vi "UpdateChannelsList.vi"(8 "error in (no error)":errorcluster, 9 "channels":string[](array[string]), 10 "asset code":string, 11 "ByteQXAPIBase in":refnum<class "ByteQXAPIBase.lvclass">) -> (0 "error out":errorcluster, 3 "ByteQXAPIBase out":refnum<class "ByteQXAPIBase.lvclass">)   [LabVIEW 2019, in "ByteQXWebAPI.lvlib" / "ByteQXAPIBase.lvclass"]
doc: "Sends the asset's available channels list"
uses:
  ByteQXAPIBase.lvclass
  Private/module.ctl
  ChannelsList_ReqData.ctl
  ByteQXAPIBase.lvclass/ByteQXAPIBase.ctl
  <vilib>/Bytelabs/ByteREST/ByteRESTClass/ByteRESTBase/RESTBase.lvclass
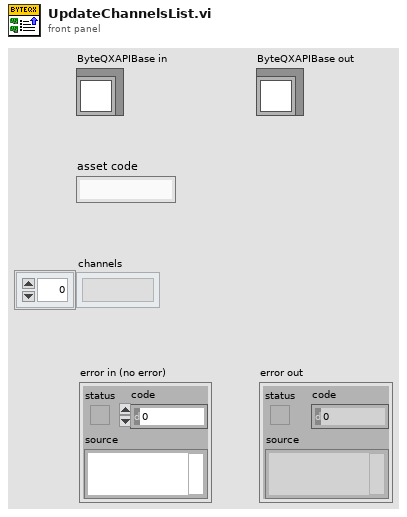
[diagram p1: front panel]
types:
  T1 = typedef "ByteQXWebAPI.lvlib/ByteQXAPIBase.lvclass/ChannelsList_ReqData.ctl" = cluster{"asset_slug":string, "fields":string[]}
  T2 = typedef "ByteQXWebAPI.lvlib/ByteQXAPIBase.lvclass/module.ctl" = enum16{"gs", "tms", "data"}
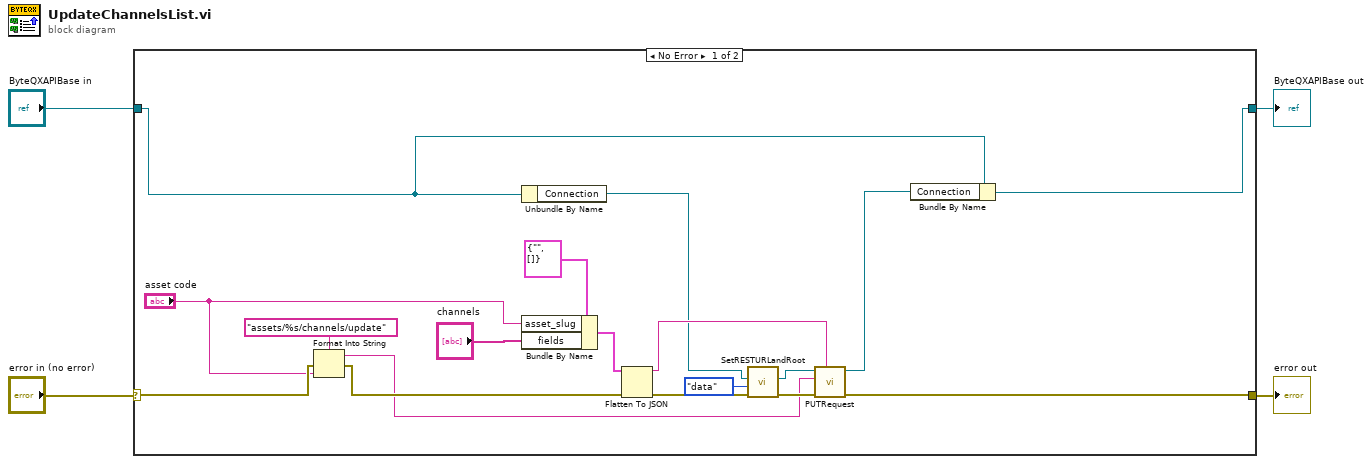
[diagram p0: block diagram]
diagram:
  n1 = case shown="No Error" "error in (no error)" {
    selector: "error in (no error)" -> [w8 w24]
    tunnel: [w20 w24] -> w3
    tunnel: [w17 w23] -> w1
    tunnel: "ByteQXAPIBase in" -> [w18 w23]
    frame No Error {
      n2 = Format Into String(format string="assets/%s/channels/update" ("Request"), error in=w8, "asset code") -> (resulting string=w5:string, error out=w7:errorcluster)  [unwired: 1 in]
      n3 = Unbundle By Name(w18) -> ("Connection"=w14:refnum<class "RESTBase.lvclass">)
      n4 = Bundle By Name(cluster=T1 {"asset_slug"="", "fields"=[]} ("Channels"), "asset_slug"="asset code", "fields"="channels") -> (w11:T1)
      n5 = Flatten To JSON(anything=w11, error in (no error)=w7) -> (JSON string=w22:string, 11:w16:errorcluster)  [unwired: 1 in]
      n6 = call "SetRESTURLandRoot.vi"("error in (no error)"=w16, "module"=module."data", "ByteREST in"=w14) -> ("error out"=w15:errorcluster, "ByteREST out"=w13:refnum<class "RESTBase.lvclass">)  [unwired: 7 in]
      n7 = call-dynamic "PUTRequest.vi"("Body in"=w22, "error in (no error)"=w15, "Request"=w5, "ByteRESTBase in"=w13) -> ("error out"=w20:errorcluster, "ByteRESTBase out"=w21:refnum<class "RESTBase.lvclass">)  [unwired: 4 in, 2 out]
      n8 = Bundle By Name(cluster=w18, "Connection"=w21) -> (w17:refnum<class "ByteQXAPIBase.lvclass">)
    }
    frame Error {
    }
  }
  "error out" <- w3
  "ByteQXAPIBase out" <- w1
